vi "DropDetectionForLinkam.vi"(5 "BCG Values":T1={"Brightness"=128.0, "Contrast"=45.0, "Gamma"=1.0} {"Brightness" min=0 max=255 step=1 format="%.2f"; "Contrast" min=1 max=89 step=1 format="%.2f"; "Gamma" min=0.1 max=10 step=0.01 format="%.2f"}, 6 "Circle Descriptor":cluster{"Min Radius":dbl, "Max Radius":dbl}={"Min Radius"=11.5499999973435, "Max Radius"=19.2499999955725}, 7 "Frame Number":u32, 8 "error in":errorcluster, 9 "Image in":T5(plugin-control)=refnum, 10 "Minimum match score":dbl=800.0, 11 "Path":path=path "T:/LabBox/Lior Segev/Debugging Freeze Software/Test-27_07_2015-13_37_03.avi") -> (0 "error out":errorcluster, 1 "Number of matches":i32, 2 "Matches (pixel)":T4(array[cluster]), 3 "Image Out":T5(plugin-control), 4 "Circles (Calibrated)":T6(array[cluster]) {"Position"."Y" format="%.2f"; "Position"."X" format="%.2f"})   [LabVIEW 2013]
uses:
  <vilib>/vision/NI_Vision_Development_Module.lvlib
  <vilib>/Analysis/NI_AALPro.lvlib
  <vilib>/Analysis/NI_AAL_SigProc.lvlib
  <resource>/objmgr/IMAQImage.rc
panel:
  out "size(s)":i32
  out "Image Size":cluster{"x":i32, "y":i32}={"x"=1600, "y"=1300}
  in  "ROI Descriptor":T2={"Global Rectangle"=[0, 958, 1278, 1060], "Contours"=[{"ID"=enum."External", "Type"=3, "Coordinates"=[0, 1198, 1600, 1300]}]} {"Contours"."Type" items=["No Selection", "Point", "Line", "Rectangle", "Oval", "Polygon", "Freehand Region", "Annulus", "Unused2", "Unused3", "Broken Line", "Freehand Line", "Rotated Rectangle"]}
  out "fractional index or x":dbl=3.330483523459592
  out "XY Graph":cluster{i32[], "dX/dt":dbl[]}[](graph)=[{[0, 1, 2, 3, 4, 5, 6, 7, 8, 9, 10, 11, 12, 13, 14, 15, 16, 17, 18, 19, 20, 21, 22, 23, 24, 25, 26, 27, 28, 29, 30, 31, 32, 33, 34, 35, 36, 37, 38, 39, 40, 41, 42, 43, 44, 45, 46, 47, 48, 49, 50, 51, 52, 53, 54, 55, 56, 57, 58, 59, 60, 61, 62, 63, 64, 65, 66, 67, 68, 69, 70, 71, 72, 73, 74, 75, 76, 77, 78, 79, 80, 81, 82, 83, 84, 85, 86, 87, 88, 89, 90, 91, 92, 93, 94, 95, 96, 97, 98, 99], "dX/dt"=[13.0, 13.0, 20.0, 247.0, 252.0, 252.0, 252.0, 254.0, 254.0, 253.0, 253.0, 253.0, 250.0, 250.0, 250.0, 254.0, 254.0, 254.0, 254.0, 254.0, 254.0, 254.0, 254.0, 254.0, 219.0, 251.0, 253.0, 253.0, 252.0, 253.0, 254.0, 252.0, 254.0, 252.0, 254.0, 253.0, 253.0, 253.0, 253.0, 255.0, 254.0, 254.0, 255.0, 254.0, 254.0, 254.0, 255.0, 255.0, 255.0, 254.0, 254.0, 252.0, 253.0, 255.0, 255.0, 255.0, 255.0, 255.0, 254.0, 254.0, 255.0, 255.0, 255.0, 253.0, 255.0, 254.0, 255.0, 255.0, 255.0, 255.0, 252.0, 255.0, 253.0, 253.0, 253.0, 254.0, 255.0, 248.0, 255.0, 255.0, 255.0, 255.0, 253.0, 255.0, 254.0, 254.0, 254.0, 254.0, 255.0, 255.0, 254.0, 254.0, 254.0, 254.0, 253.0, 255.0, 254.0, 254.0, 252.0, 252.0]}, {[0, 1, 2, 3, 4, 5, 6, 7, 8, 9, 10, 11, 12, 13, 14, 15, 16, 17, 18, 19, 20, 21, 22, 23, 24, 25, 26, 27, 28, 29, 30, 31, 32, 33, 34, 35, 36, 37, 38, 39, 40, 41, 42, 43, 44, 45, 46, 47, 48, 49, 50, 51, 52, 53, 54, 55, 56, 57, 58, 59, 60, 61, 62, 63, 64, 65, 66, 67, 68, 69, 70, 71, 72, 73, 74, 75, 76, 77, 78, 79, 80, 81, 82, 83, 84, 85, 86, 87, 88, 89, 90, 91, 92, 93, 94, 95, 96, 97, 98, 99], "dX/dt"=[6.5, 3.5, 117.0, 116.0, 2.5, 0.0, 1.0, 1.0, -0.5, -0.5, 0.0, -1.5, -1.5, 0.0, 2.0, 2.0, 0.0, 0.0, 0.0, 0.0, 0.0, 0.0, 0.0, -17.5, -1.5, 17.0, 1.0, -0.5, 0.0, 1.0, -0.5, 0.0, 0.0, 0.0, 0.5, -0.5, 0.0, 0.0, 1.0, 0.5, -0.5, 0.5, 0.0, -0.5, 0.0, 0.5, 0.5, 0.0, -0.5, -0.5, -1.0, -0.5, 1.5, 1.0, 0.0, 0.0, 0.0, -0.5, -0.5, 0.5, 0.5, 0.0, -1.0, 0.0, 0.5, 0.0, 0.5, 0.0, 0.0, -1.5, 0.0, 0.5, -1.0, 0.0, 0.5, 1.0, -3.0, 0.0, 3.5, 0.0, 0.0, -1.0, 0.0, 0.5, -0.5, 0.0, 0.0, 0.5, 0.5, -0.5, -0.5, 0.0, 0.0, -0.5, 0.5, 0.5, -0.5, -1.0, -1.0, -126.0]}]
  in  "Annulus":T3 {"End Angle" min=-90.0 max=90.0 step=1.0 format="%.2f"; "Start Angle" min=-90.0 max=90.0 step=1.0 format="%.2f"; "Center X" scale=0.0..1024.0}
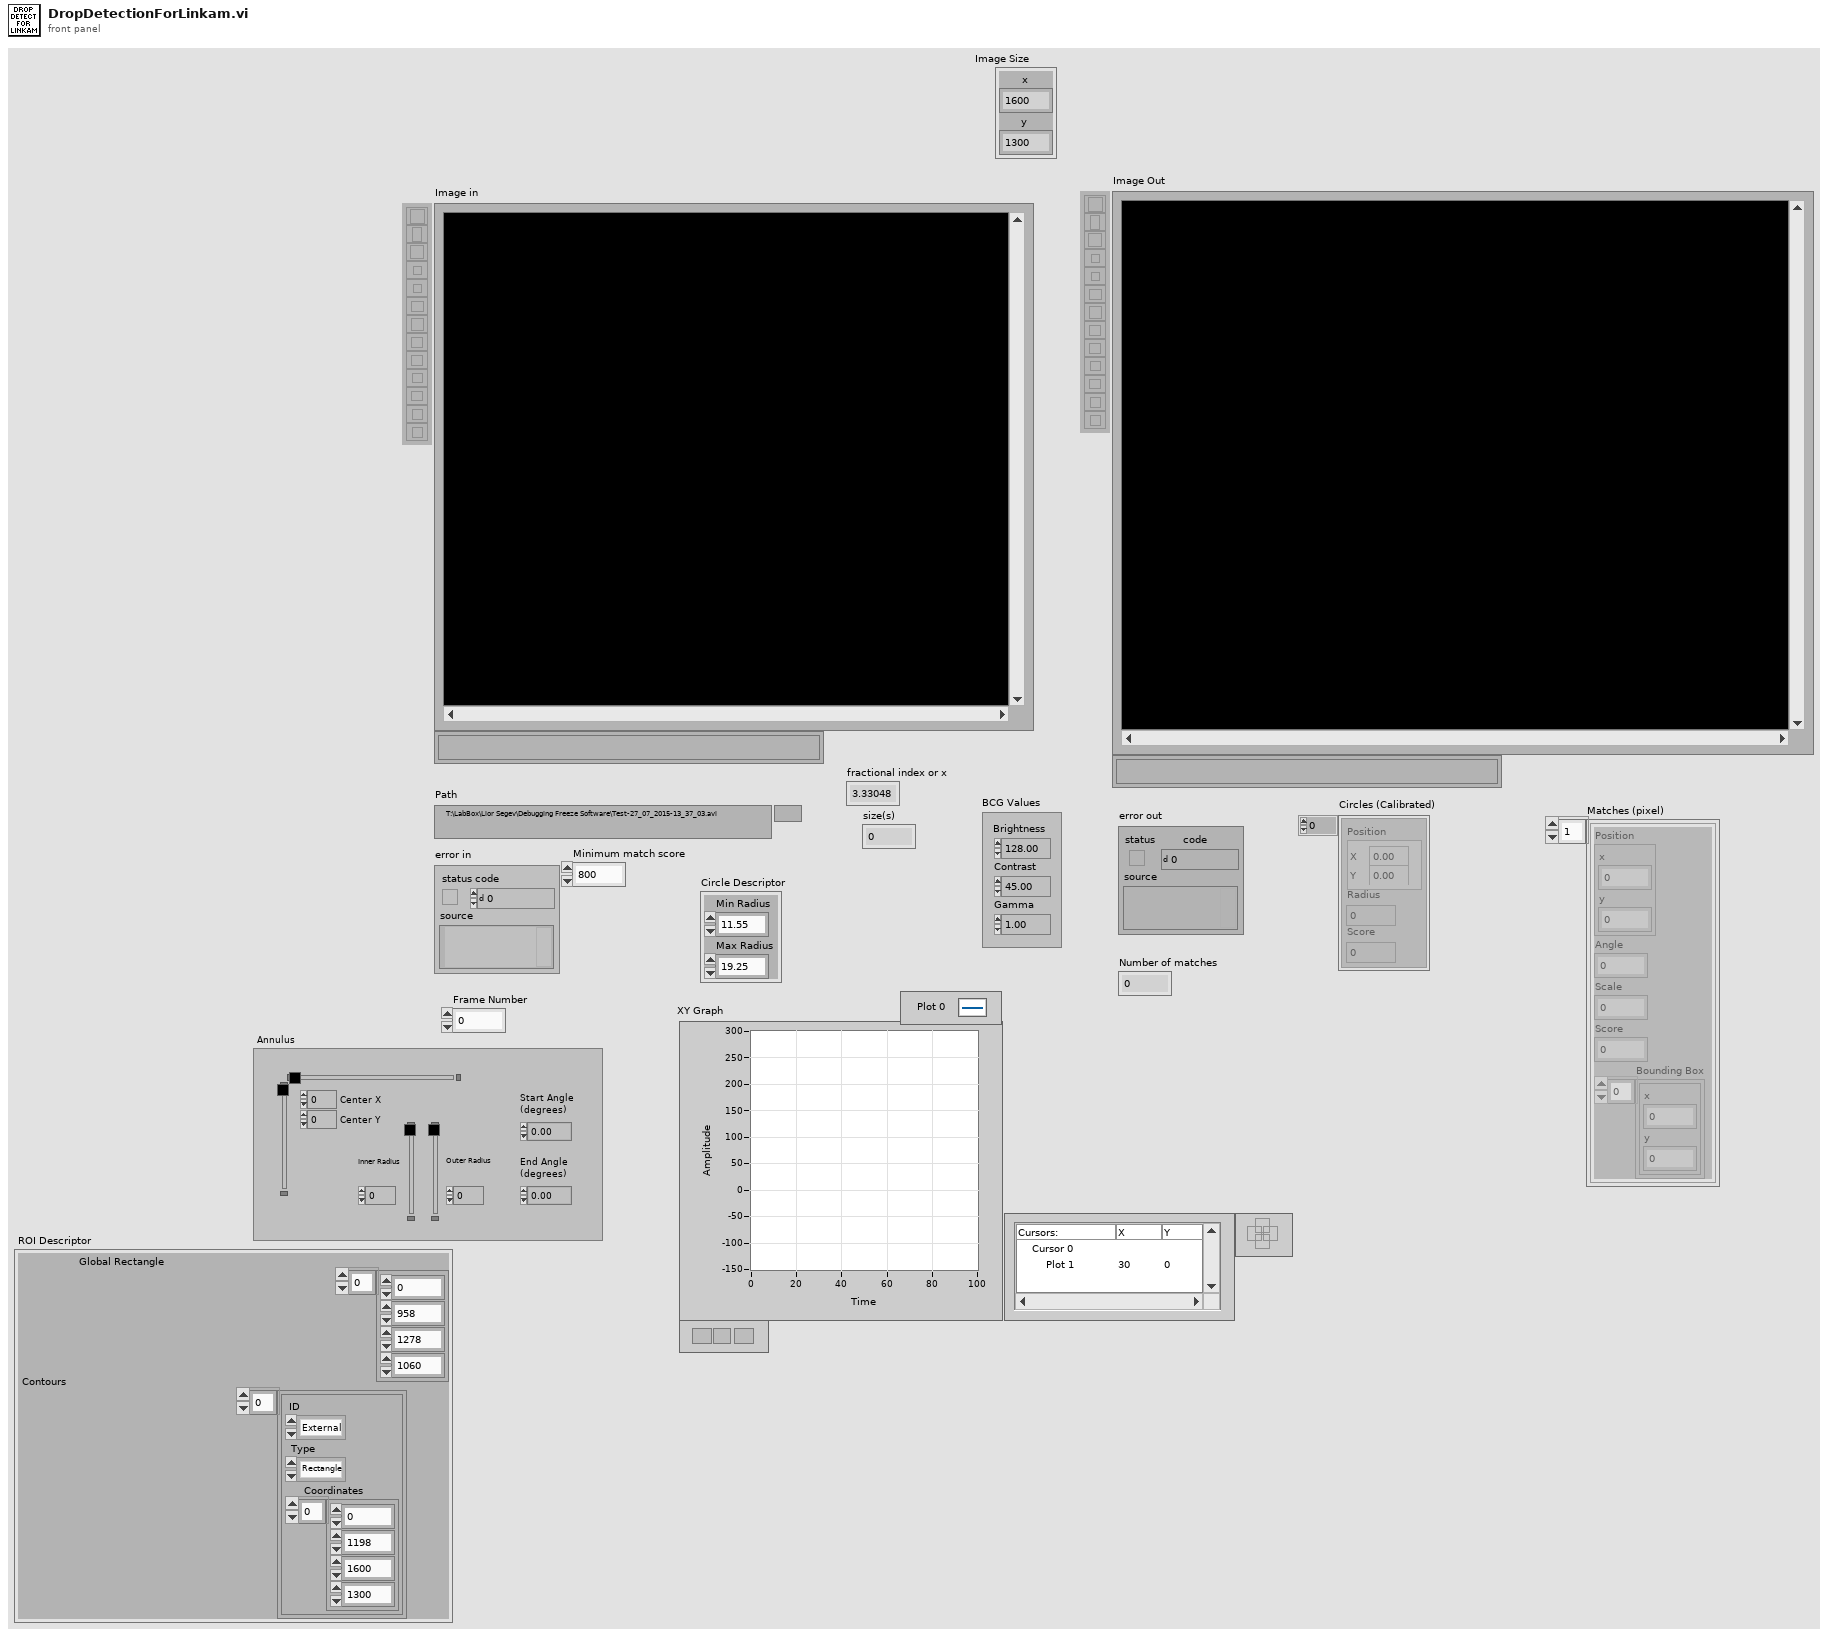
[diagram p1: front panel]
types:
  T1 = cluster{"Brightness":sgl, "Contrast":sgl, "Gamma":sgl}
  T2 = cluster{"Global Rectangle":i32[], "Contours":cluster{"ID":enum32{"External", "Internal"}, "Type":u32, "Coordinates":i32[]}[]}
  T3 = typedef "IMAQ Circle" = cluster{"Center X":i32, "Center Y":i32, "Inner Radius":i32, "Outer Radius":i32, "Start Angle":dbl, "End Angle":dbl}
  T4 = cluster{"Position":cluster{"x":sgl, "y":sgl}, "Angle":sgl, "Scale":sgl, "Score":sgl, "Bounding Box":cluster{"x":sgl, "y":sgl}[]}[]
  T5 = typedef "IMAQ Image.ctl" = refnum<image>
  T6 = cluster{"Position":cluster{"X":sgl, "Y":sgl}, "Radius":dbl, "Score":dbl}[]
  T7 = cluster{"Extraction Mode":u32, "Edge Threshold":i32, "Edge Filter Size":u32, "Min Length":i32, "Row Search Step Size":i32, "Col Search Step Size":i32, "Max Endpoint Gap":i32, "Closed":bool, "Subpixel":bool}
  T8 = cluster{"Rotation":bool, "Scale":bool, "Occlusion":bool, "Range Settings":cluster{"Match Constraints":u32, "Min":dbl, "Max":dbl}[]}
  T9 = typedef "IMAQ AVI2 Refnum.ctl" = refnum<k20>
  T10 = cluster{"ID":enum32{"External", "Internal"}, "Type":u32, "Coordinates":i32[]}[]
  T11 = cluster{"ID":enum32{"External", "Internal"}, "Type":u32, "Coordinates":i32[]}
  T12 = typedef "ROI Descriptor" = cluster{"Global Rectangle":i32[], "Contours":cluster{"ID":enum32{"External", "Internal"}, "Type":u32, "Coordinates":i32[]}[]}
  T13 = cluster{"Min":sgl, "Max":sgl, "Mean":sgl, "Std Dev":sgl, "Count":i32}
  T14 = cluster{"Position":cluster{"X":sgl, "Y":sgl}, "Radius":dbl, "Score":dbl}
  T15 = cluster{"Position":cluster{"x":sgl, "y":sgl}, "Angle":sgl, "Scale":sgl, "Score":sgl, "Bounding Box":cluster{"x":sgl, "y":sgl}[]}
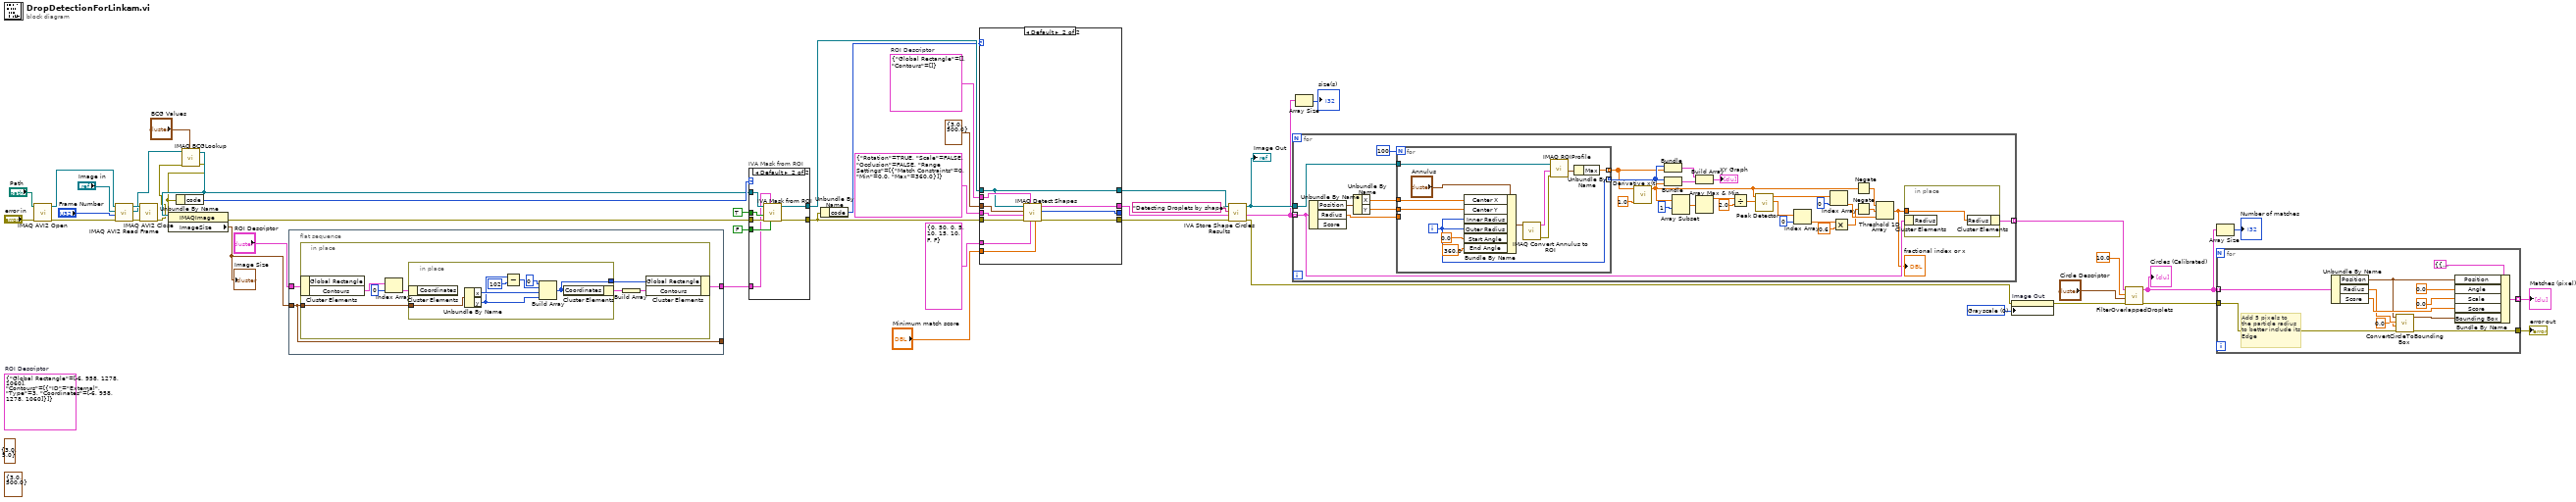
[diagram p0: block diagram]
diagram:
  (unwired) cluster{"Min Radius":dbl, "Max Radius":dbl} {"Min Radius"=3.0, "Max Radius"=500.0} ("Circle Descriptor")
  (unwired) cluster{"Min Radius":dbl, "Max Radius":dbl} {"Min Radius"=3.0, "Max Radius"=5.0} ("Circle Descriptor")
  w33 = u32 0 items=["Grayscale", "Binary", "Gradient", "Rainbow", "Temperature", "User Defined"] ("Palette")
  w41 = T2 {"Global Rectangle"=[], "Contours"=[]}  # ROI Descriptor
  (unwired) T2 {"Global Rectangle"=[-6, 958, 1278, 1060], "Contours"=[{"ID"=enum."External", "Type"=3, "Coordinates"=[-6, 958, 1278, 1060]}]}  # ROI Descriptor
  n1 = call "IMAQ AVI2 Open"("error in (no error)"="error in", "AVI File Path"="Path") -> ("error out"=w31:errorcluster, "AVI Refnum"=w30:T9)  [unwired: 8 in]
  n2 = call "IMAQ AVI2 Read Frame"("error in (no error)"=w31, "Frame Number"="Frame Number", "Image"="Image in", "AVI Refnum"=w30) -> ("error out"=w29:errorcluster, "Image Out"=w5:T5, "AVI Refnum (duplicate)"=w28:T9)  [unwired: 5 in]
  n3 = call "IMAQ AVI2 Close"("error in (no error)"=w29, "AVI Refnum"=w28) -> ("error out"=w3:errorcluster)  [unwired: 9 in]
  n4 = call "IMAQ BCGLookup"("Image Src"=w5, "BCG Values"="BCG Values", "error in (no error)"=w3) -> ("Image Dst Out"=w4:T5, "error out"=w2:errorcluster)  [unwired: 4 in]
  n5 = property class="IMAQImage"(reference=w4, error in=w2) -> (error out=w11:errorcluster, "ImageSize"=w10:cluster{"x":i32, "y":i32})  [unwired: 1 out]
  "Image Size" <- w10
  n6 = Unbundle By Name(w2) -> ("code"=w44:i32)
  n7 = flat-sequence {
    tunnel: [w48] -> _
    tunnel: w10 -> [w48]
    tunnel: "ROI Descriptor" -> [w49]
    tunnel: [w47] -> w8
    frame #0 {
      n8 = in-place {
        in-place-border: w48 -> [w53]
        n9 = in-place-cluster #1(w49) -> ("Contours"=w55:T10)  [unwired: 1 out]
        n10 = Index Array(array=w55, index=0) -> (element=w54:T11)
        n11 = in-place {
          in-place-border: w53 -> [w62]
          in-place-border: [w57] -> w50
          n12 = in-place-cluster #2(w54) -> ()  [unwired: 1 out]
          n13 = Unbundle By Name(w62) -> ("x"=w61:i32, "y"=w59:i32)
          n14 = Subtract(x=w59, y=102) -> (x-y=w58:i32)
          n15 = Build Array(0 ("element"), w58, w61, w59) -> (w57:i32[])
          n16 = in-place-cluster #2("Coordinates"=w57) -> (w52:T11)
        }
        n17 = Build Array(w52) -> (w51:T10)
        n18 = in-place-cluster #1("Global Rectangle"=w50, "Contours"=w51) -> (w47:T2)
      }
    }
  }
  n19 = case "IVA Mask from ROI" shown="Default" w44 {
    tunnel: FALSE ("Shrink") -> [_ w71]
    tunnel: w4 -> [w64 w70]
    tunnel: w11 -> [_ w69]
    tunnel: [_ w68] -> w36
    tunnel: [w64 w67] -> w39
    tunnel: TRUE ("Out / In") -> [_ w66]
    tunnel: w8 -> [_ w65]
    frame -1074396199, -1074396198 {
      # "Discard\nCoordinate\nSystem\nError"
    }
    frame Default {
      n20 = call <vilib>:"IVA Mask from ROI.vi"("Shrink"=w71, "ROI Descriptor"=w65, "error in (no error)"=w69, "Out / In"=w66, "Image Src"=w70) -> ("error out"=w68:errorcluster, "Image Out"=w67:T5)  [unwired: 5 out]
    }
  }
  n21 = Unbundle By Name(w36) -> ("code"=w35:i32)
  n22 = case shown="Default" w35 {
    tunnel: w36 -> [_ w82]
    tunnel: [_ w81] -> _
    tunnel: T8 {"Rotation"=TRUE, "Scale"=FALSE, "Occlusion"=FALSE, "Range Settings"=[{"Match Constraints"=0, "Min"=0.0, "Max"=360.0}]} ("Match Options") -> [_ w80]
    tunnel: T7 {"Extraction Mode"=0, "Edge Threshold"=50, "Edge Filter Size"=0, "Min Length"=5, "Row Search Step Size"=10, "Col Search Step Size"=15, "Max Endpoint Gap"=10, "Closed"=FALSE, "Subpixel"=FALSE} ("Curve Parameters") -> [_ w79]
    tunnel: "Minimum match score" -> [_ w78]
    tunnel: cluster{"Min Radius":dbl, "Max Radius":dbl} {"Min Radius"=3.0, "Max Radius"=500.0} ("Circle Descriptor") -> [_ w77]
    tunnel: w41 -> [_ w76]
    tunnel: [_ w75] -> w40
    tunnel: w39 -> [w72 w73]
    tunnel: [_ w74] -> w38
    tunnel: [w72 w73] -> w34
    frame -1074396199, -1074396198 {
      # "Discard Coordinate\nSystem Error"
    }
    frame Default {
      n23 = call-poly "IMAQ Detect Shapes"("Minimum match score"=w78, "Curve Parameters"=w79, "ROI Descriptor"=w76, "error in (no error)"=w82, "Match Options"=w80, "Circle Descriptor"=w77, "Image"=w73) -> ("error out"=w74:errorcluster, "Number of Matches Returned"=w81:i32, "Circles"=w75:T6)  [unwired: 2 out]
    }
  }
  n24 = call <vilib>:"IVA Store Shape Circles Results.vi"("error in (no error)"=w38, "Circles"=w40, "Step Name"="Detecting Droplets by shape", "Image in"=w34) -> ("error out"=w32:errorcluster, "Circles (Calibrated)"=w7:T6, "Image dup"=w14:T5)  [unwired: 5 out]
  "Image Out" <- w14
  n25 = for {
    tunnel: w14 -> [w113]
    tunnel: w7 -> [w94] mode=indexing
    tunnel: [w93] -> w13 mode=indexing
    n26 = Unbundle By Name(w94) -> ("Position"=w112:cluster{"X":sgl, "Y":sgl}, "Radius"=w95:dbl)  [unwired: 1 out]
    n27 = Unbundle By Name(w112) -> ("X"=w111:sgl, "Y"=w110:sgl)
    n28 = for {
      N: 100 -> [_]
      tunnel: w113 -> [w125]
      tunnel: w95 -> [_]
      tunnel: w111 -> [w122]
      tunnel: w110 -> [w121]
      tunnel: [w117] -> w107 mode=indexing
      tunnel: [w115] -> w108 mode=indexing
      i -> [w115]
      n29 = Bundle By Name(cluster="Annulus", "Center X"=w122, "Center Y"=w121, "Inner Radius"=w115, "Outer Radius"=w115, "Start Angle"=0.0, "End Angle"=360.0) -> (w120:T3)
      n30 = call "IMAQ Convert Annulus to ROI"("Annulus"=w120) -> ("error out"=w119:errorcluster, "ROI Descriptor"=w126:T12)  [unwired: 8 in]
      n31 = call "IMAQ ROIProfile"("error in (no error)"=w119, "ROI Descriptor"=w126, "Image"=w125) -> ("ROI Pixel Statistics"=w118:T13)  [unwired: 1 in, 4 out]
      n32 = Unbundle By Name(w118) -> ("Max"=w117:sgl)
    }
    n33 = call <vilib>:"Derivative x(t).vi"("dt"=1.0, "X"=w107) -> ("dX/dt"=w87:dbl[])  [unwired: 8 in, 1 out]
    n34 = Bundle(w108, w107) -> (w106:cluster{i32[], sgl[]})  [unwired: 1 in]
    n35 = Bundle(w108, "dX/dt"=w87) -> (w105:cluster{i32[], "dX/dt":dbl[]})  [unwired: 1 in]
    n36 = Array Subset(array=w87, index=1) -> (w101:dbl[])  [unwired: 1 in]
    n37 = Build Array(w106, w105) -> (→"XY Graph":cluster{i32[], "dX/dt":dbl[]}[])
    n38 = Array Max & Min(array=w101) -> (max value=w100:dbl)  [unwired: 3 out]
    n39 = Divide(x=w100, y=2.0) -> (x/y=w98:dbl)
    n40 = call <vilib>:"Peak Detector.vi"("threshold"=w98, "X"=w87) -> ("Amplitudes"=w90:dbl[], "Locations"=w97:dbl[])  [unwired: 5 in, 3 out]
    n41 = Index Array(array=w90, index=0) -> (element=w88:dbl)
    n42 = Index Array(array=w97, index=0) -> (element=w92:dbl)
    n43 = Multiply(x=w88, y=0.6) -> (x*y=w85:dbl)
    n44 = Negate(x=w87) -> (-x=w86:dbl[])
    n45 = Negate(x=w85) -> (-x=w84:dbl)
    n46 = Threshold 1D Array(1:w92, 2:w84, 3:w86) -> (0:w83:dbl)
    "fractional index or x" <- w83
    n47 = in-place {
      in-place-border: w83 -> [w114]
      n48 = in-place-cluster #3(w94) -> ()  [unwired: 1 out]
      n49 = in-place-cluster #3("Radius"=w114) -> (w93:T14)
    }
  }
  n50 = Array Size(array=w7) -> (size(s)=→"size(s)":i32)
  n51 = property on="Image Out" class="ImageControl"(error in=w32, "Palette:Palette Type"=w33) -> (error out=w19:errorcluster)  [unwired: 1 in, 1 out]
  n52 = call "FilterOverlappedDroplets.vi"("error in (no error)"=w19, "Circle Descriptor"="Circle Descriptor", "Threshold (pixels)"=10.0, "Circles (Calibrated)"=w13) -> ("error out"=w16:errorcluster, "Circles (Calibrated) 2"=w12:T6)  [unwired: 6 in]
  "Circles (Calibrated)" <- w12
  n53 = Array Size(array=w12) -> (size(s)=→"Number of matches":i32)
  n54 = for {
    tunnel: w12 -> [w137] mode=indexing
    tunnel: [w133] -> w21 mode=indexing
    tunnel: w16 -> [w128]
    tunnel: [w127] -> w15
    # "Add 5 pixels to\nthe particle radius \nto better include its\nEdge"
    n55 = Unbundle By Name(w137) -> ("Position"=w131:cluster{"X":sgl, "Y":sgl}, "Radius"=w130:dbl, "Score"=w136:dbl)
    n56 = call "ConvertCircleToBoundingBox.vi"("error in (no error)"=w128, "InflateBoxbyPixelNo"=0.0 ("y"), "Radius"=w130, "Position"=w131) -> ("error out"=w127:errorcluster, "Bounding Box"=w132:cluster{"x":sgl, "y":sgl}[])  [unwired: 6 in]
    n57 = Bundle By Name(cluster=T15 {"Position"={"x"=0.0, "y"=0.0}, "Angle"=0.0, "Scale"=0.0, "Score"=0.0, "Bounding Box"=[]} ("element"), "Position"=w131, "Angle"=sgl 0.0, "Scale"=sgl 0.0, "Score"=w136, "Bounding Box"=w132) -> (w133:T15)
  }
  "error out" <- w15
  "Matches (pixel)" <- w21
